vi "tls init.vi"(8 "error in":errorcluster) -> (0 "error out":errorcluster)   [LabVIEW 2016, in "lv tls dll.lvlib"]
uses:
  lv tls dll.lvlib
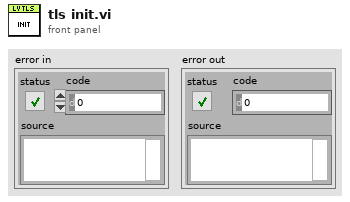
[diagram p1: front panel]
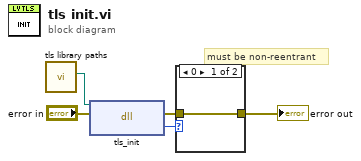
[diagram p0: block diagram]
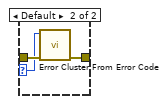
[diagram p2: hidden frame]
diagram:
  # "must be non-reentrant"
  n1 = call "tls library paths.vi"() -> ("libtls"=w5:path)  [unwired: 8 in, 3 out]
  n2 = dll-call lib="C:/Users/IEUser/Desktop/tlssimple/libtls-15.dll" fn="tls_init"(path in=w5, error in="error in") -> (error out=w3:errorcluster, "return"=w1:i32)  [unwired: 1 in, 1 out]
  n3 = case shown="0" w1 {
    selector: w1 -> [_ w7]
    tunnel: w3 -> [w6 w9]
    tunnel: [w6 w8] -> w2
    frame 0 {
    }
    frame Default {
      n4 = call <vilib>:"Error Cluster From Error Code.vi"("error in (no error)"=w9, "error code (0)"=w7) -> ("error out"=w8:errorcluster)  [unwired: 7 in]
    }
  }
  "error out" <- w2
